vi "Global res manuali.vi"() -> ()   [LabVIEW 2019]
panel:
  out "Ins resistomat manuale":bool
  out "Ins res meter manuale":bool
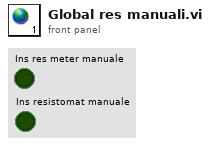
[diagram p1: front panel]
diagram:
